vi "Centered_Text.vi"(4 "String":string) -> (1 "new picture":picture)   [LabVIEW 2023]
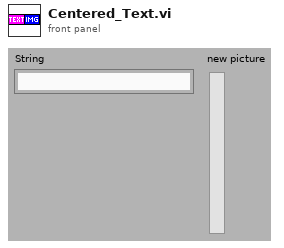
[diagram p1: front panel]
types:
  T1 = cluster{"Font Name:":string, "Size":i16, "Strikeout?":bool, "Italic?":bool, "Underline?":bool, "Outline?":bool, "Shadow?":bool, "Bold?":bool}
  T2 = enum16{"User-specified Font", "Application Font", "System Font", "Dialog Font"}
  T3 = enum16{"None", "Stacked", "Clockwise", "Counterclockwise"}
  T4 = cluster{"horizontal":enum16{"left", "center", "right"}, "vertical":enum16{"top", "center", "bottom"}}
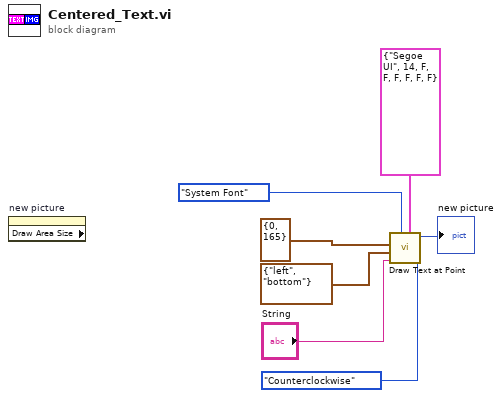
[diagram p0: block diagram]
diagram:
  n1 = property on="new picture" class="Pict" props=["Draw Area Size"]() -> ()  [unwired: 2 in, 3 out]
  n2 = call <vilib>:"Draw Text at Point.vi"("text orientation"=T3."Counterclockwise", "[user-specified font]"=T1 {"Font Name:"="Segoe UI", "Size"=14, "Strikeout?"=FALSE, "Italic?"=FALSE, "Underline?"=FALSE, "Outline?"=FALSE, "Shadow?"=FALSE, "Bold?"=FALSE}, "desired font(Application)"=T2."System Font", "text"="String", "alignment(left, top)"=T4 {"horizontal"=enum."left", "vertical"=enum."bottom"}, "origin"=cluster{"x":i16, "y":i16} {"x"=0, "y"=165}) -> ("new picture"=→"new picture":picture)  [unwired: 4 in, 1 out]
